vi "Set Protocol Data.vi"(7 "Operation":T1, 8 "error in (no error)":errorcluster, 10 "Protocols.lvlib:Protocol Parent.lvclass":refnum<class "Protocol Parent.lvclass">, 11 "Listener In.lvclass":refnum<class "Listener.lvclass"> caption="Listener") -> (0 "error out":errorcluster, 3 "Listener Out.lvclass":refnum<class "Listener.lvclass">)   [LabVIEW 2019, in "Listener.lvclass"]
uses:
  Listener.lvclass
  Protocol Parent/Protocol Parent.lvclass
  ListenerClassControls/Operation.ctl
  AK TCP/AK TCP.lvclass
  D:/GitRepository/niveristand-instrument-addon-classes/Source/Protocols/TCP/TCP.lvclass
  ListenerClassControls/AK TCP Data Structure.ctl
  ListenerClassControls/Protocol.ctl
  TCP/TCP.lvclass/TCP.ctl
  TCP/TCP.lvclass
  ListenerClassControls/TCP Data Structure.ctl
  UDP/UDP.lvclass
  ListenerClassControls/UDP Data Structure.ctl
  UDP/UDP.lvclass/UDP.ctl
  TCP/Data Access/Read IP Address.vi
  TCP/Data Access/Read Port.vi
  UDP/Data Access/Read Target IP Address.vi
  UDP/Data Access/Read Local Port.vi
  UDP/Data Access/Read Local IP Address.vi
  UDP/Data Access/Read Target Port.vi
  Constants.vi
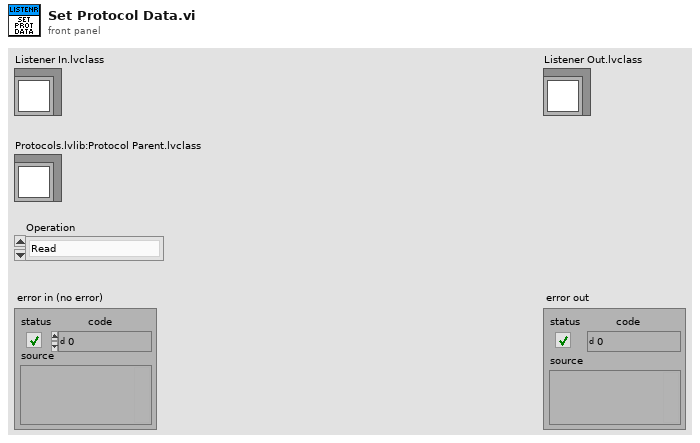
[diagram p1: front panel]
types:
  T1 = typedef "Listener.lvclass/Operation.ctl" = enum16{"Read", "Write"}
  T2 = typedef "Listener.lvclass/Protocol.ctl" = enum16{"RS-XXX", "AK RS-XXX", "VISA", "TCPIP", "AK TCPIP", "UDP", "GPIB ConvBox"}
  T3 = typedef "Listener.lvclass/AK TCP Data Structure.ctl" = cluster{"TCP|IP connection ID":refnum<k5>, "IP Address":string, "Port":u16, "Data":string, "Current Command Code":string}
  T4 = typedef "Listener.lvclass/TCP Data Structure.ctl" = cluster{"TCP|IP connection ID":refnum<k5>, "IP Address":string, "Port":u16, "Data":string}
  T5 = typedef "Listener.lvclass/UDP Data Structure.ctl" = cluster{"UDP connection ID":refnum<k16>, "Local Address":string, "Local Port":u16, "Target IP Address":string, "Target Port":u16, "Data":string}
  T6 = typedef "Protocols.lvlib/Protocol Parent.lvclass/Base Protocol Type.ctl" = enum16{"RS-XXX", "VISA", "TCPIP", "UDP", "GPIB ConvBox"}
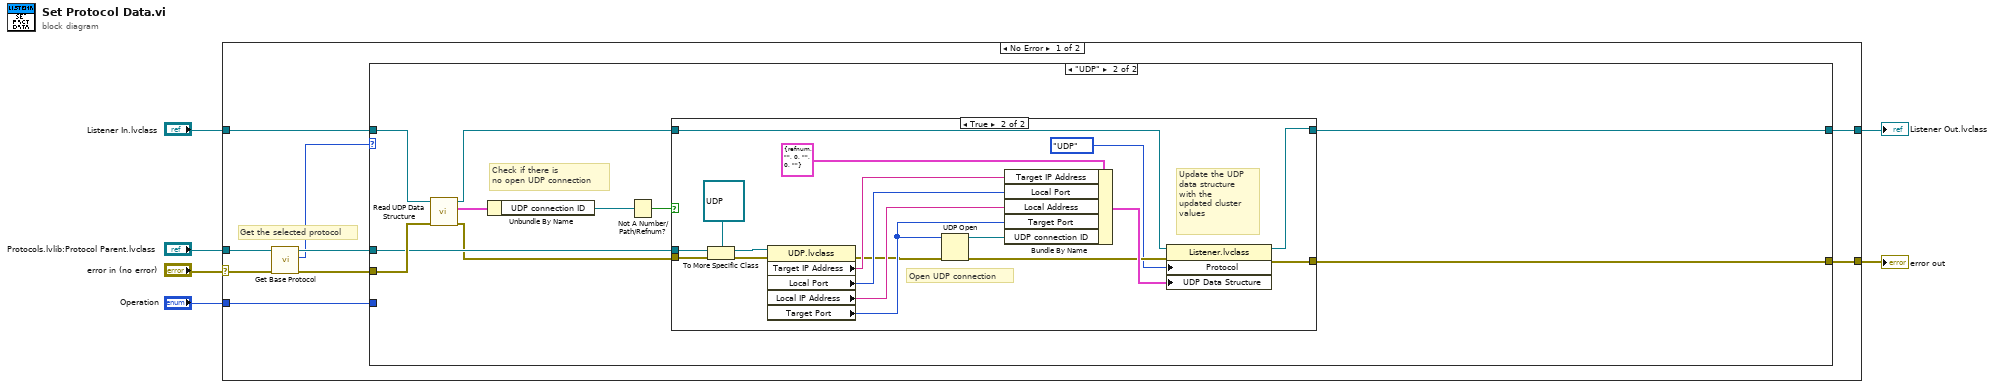
[diagram p0: block diagram]
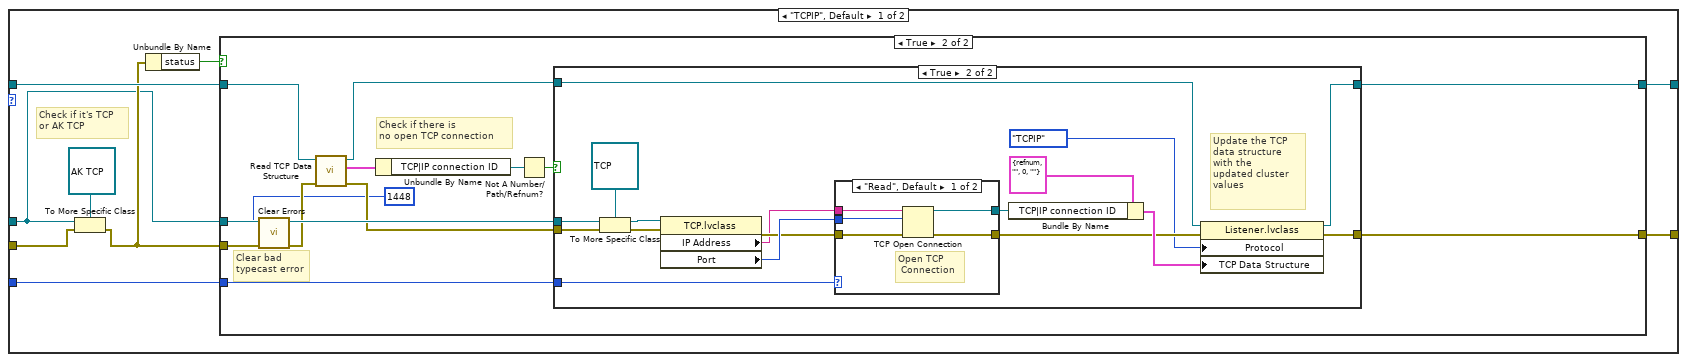
[diagram p2: hidden frame]
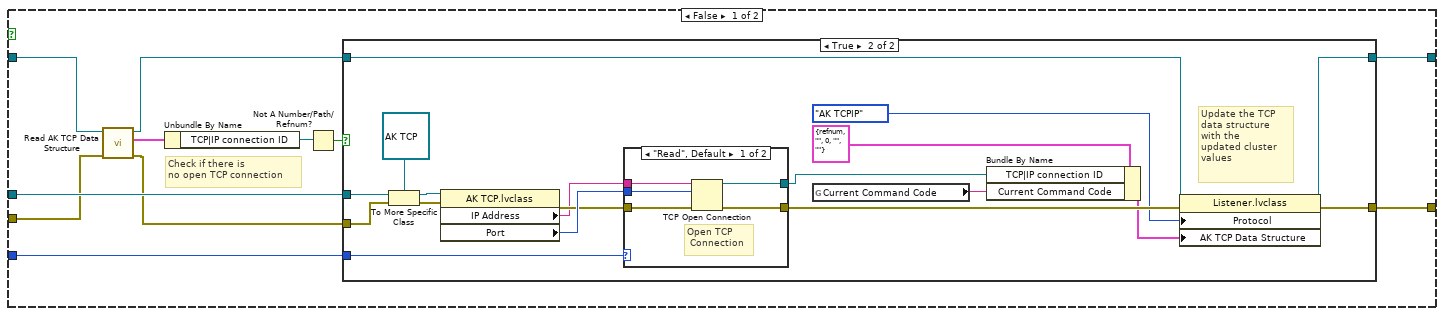
[diagram p3: hidden frame]
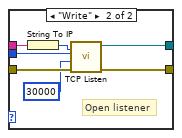
[diagram p5: hidden frame]
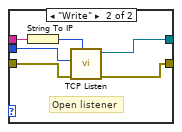
[diagram p7: hidden frame]
diagram:
  n1 = case shown="No Error" "error in (no error)" {
    selector: "error in (no error)" -> [w13 w142]
    tunnel: [w12 w142] -> w5
    tunnel: "Protocols.lvlib:Protocol Parent.lvclass" -> [w14 _]
    tunnel: "Listener In.lvclass" -> [w11 w141]
    tunnel: [w8 w141] -> w2
    tunnel: "Operation" -> [w7 _]
    frame No Error {
      # "Get the selected protocol"
      n2 = call-dynamic "Get Base Protocol.vi"("error in (no error)"=w13, "Protocol Parent in"=w14) -> ("error out"=w10:errorcluster, "Protocol out"=w9:T6, "Protocol Parent out"=w15:refnum<class "Protocol Parent.lvclass">)  [unwired: 7 in]
      n3 = case shown="\"UDP\"" w9 {
        tunnel: w15 -> [w16 w114]
        tunnel: w10 -> [w20 w116]
        tunnel: [w23 w119] -> w12
        tunnel: w11 -> [w22 w115]
        tunnel: [w24 w120] -> w8
        tunnel: w7 -> [w21 _]
        frame "TCPIP", Default {
          # "Check if it's TCP \nor AK TCP"
          n4 = To More Specific Class(target class=refnum<class "AK TCP.lvclass"> refnum ("Protocols.lvlib:AK TCP.lvclass"), reference=w16, error in=w20) -> (error out=w19:errorcluster)  [unwired: 1 out]
          n5 = Unbundle By Name(w19) -> ("status"=w18:bool)
          n6 = case shown="True" w18 {
            tunnel: w16 -> [w35 w80]
            tunnel: [w34 w79] -> w24
            tunnel: [w33 w78] -> w23
            tunnel: w22 -> [w30 w76]
            tunnel: w19 -> [w28 w75]
            tunnel: w21 -> [w31 w70]
            frame False {
              # "Check if there is \nno open TCP connection"
              n7 = call-dynamic "Read AK TCP Data Structure.vi"("error in (no error)"=w28, "Listener in"=w30) -> ("error out"=w27:errorcluster, "TCP|IP Data Structure"=w26:T3, "Listener out"=w29:refnum<class "Listener.lvclass">)  [unwired: 7 in]
              n8 = Unbundle By Name(w26) -> ("TCP|IP connection ID"=w25:refnum<k5>)
              n9 = Not A Number/Path/Refnum?(number/path/refnum=w25) -> (NaN/Path/Refnum?=w32:bool)
              n10 = case shown="True" w32 {
                tunnel: w35 -> [_ w55]
                tunnel: [w37 w52] -> w34
                tunnel: [w36 w51] -> w33
                tunnel: w27 -> [w36 w50]
                tunnel: w29 -> [w37 w49]
                tunnel: w31 -> [_ w48]
                frame False {
                }
                frame True {
                  # "Update the TCP \ndata structure\nwith the\nupdated cluster\nvalues"
                  n11 = To More Specific Class(target class=refnum<class "AK TCP.lvclass"> refnum ("Protocols.lvlib:AK TCP.lvclass"), reference=w55, error in=w50) -> (specific class reference=w54:refnum<class "AK TCP.lvclass">, error out=w53:errorcluster)
                  n12 = property class="AK TCP.lvclass"(reference=w54, error in=w53) -> (error out=w46:errorcluster, "IP Address"=w45:string, "Port"=w47:u16)  [unwired: 1 out]
                  n13 = case shown="\"Read\", Default" w48 {
                    tunnel: w47 -> [w60 w62]
                    tunnel: w46 -> [w59 w67]
                    tunnel: w45 -> [w58 w66]
                    tunnel: [w57 w63] -> w44
                    tunnel: [w56 w64] -> w43
                    frame "Read", Default {
                      # "Open TCP\n Connection"
                      n14 = TCP Open Connection(address=w58, remote port or service name=w60, error in (no error)=w59) -> (connection ID=w56:refnum<k5>, error out=w57:errorcluster)  [unwired: 2 in]
                    }
                    frame "Write" {
                      # "Open listener"
                      n15 = String To IP(1:w66) -> (0:w65:u32)
                      n16 = call <vilib>:"TCP Listen.vi"("net address"=w65, "error in (no error)"=w67, "timeout ms (wait forever: -1)"=30000, "port"=w62) -> ("error out"=w63:errorcluster, "connection ID"=w64:refnum<k5>)  [unwired: 3 in, 3 out]
                    }
                  }
                  n17 = global read "Constants.vi" "Current Command Code"() -> (w38:string)
                  n18 = Bundle By Name(cluster=T3 {"TCP|IP connection ID"=refnum, "IP Address"="", "Port"=0, "Data"="", "Current Command Code"=""} ("TCP|IP Data Structure"), "TCP|IP connection ID"=w43, "Current Command Code"=w38) -> (w40:T3)
                  n19 = property class="Listener.lvclass"(reference=w49, error in=w44, "Protocol"=Protocol."AK TCPIP", "AK TCP Data Structure"=w40) -> (reference out=w52:refnum<class "Listener.lvclass">, error out=w51:errorcluster)
                }
              }
            }
            frame True {
              # "Clear bad \ntypecast error"
              # "Check if there is \nno open TCP connection"
              n20 = call <vilib>:"Clear Errors.vi"("error in (no error)"=w75, "specific error code to clear (0: all)"=1448) -> ("error out"=w69:errorcluster)  [unwired: 4 in, 1 out]
              n21 = call-dynamic "Read TCP Data Structure.vi"("error in (no error)"=w69, "Listener in"=w76) -> ("error out"=w74:errorcluster, "TCP|IP Data Structure"=w73:T4, "Listener out"=w72:refnum<class "Listener.lvclass">)  [unwired: 7 in]
              n22 = Unbundle By Name(w73) -> ("TCP|IP connection ID"=w77:refnum<k5>)
              n23 = Not A Number/Path/Refnum?(number/path/refnum=w77) -> (NaN/Path/Refnum?=w71:bool)
              n24 = case shown="True" w71 {
                tunnel: w80 -> [_ w98]
                tunnel: [w82 w94] -> w79
                tunnel: [w81 w92] -> w78
                tunnel: w74 -> [w81 w91]
                tunnel: w72 -> [w82 w90]
                tunnel: w70 -> [_ w89]
                frame False {
                }
                frame True {
                  # "Update the TCP \ndata structure\nwith the\nupdated cluster\nvalues"
                  n25 = To More Specific Class(target class=refnum<class "TCP.lvclass"> refnum ("Protocols.lvlib:TCP.lvclass"), reference=w98, error in=w91) -> (specific class reference=w97:refnum<class "TCP.lvclass">, error out=w96:errorcluster)
                  n26 = property class="TCP.lvclass"(reference=w97, error in=w96) -> (error out=w87:errorcluster, "IP Address"=w86:string, "Port"=w88:u16)  [unwired: 1 out]
                  n27 = case shown="\"Read\", Default" w89 {
                    tunnel: w88 -> [w104 w109]
                    tunnel: w87 -> [w103 w110]
                    tunnel: w86 -> [w102 w108]
                    tunnel: [w101 w105] -> w85
                    tunnel: [w100 w106] -> w84
                    frame "Read", Default {
                      # "Open TCP\n Connection"
                      n28 = TCP Open Connection(address=w102, remote port or service name=w104, error in (no error)=w103) -> (connection ID=w100:refnum<k5>, error out=w101:errorcluster)  [unwired: 2 in]
                    }
                    frame "Write" {
                      # "Open listener"
                      n29 = String To IP(1:w108) -> (0:w107:u32)
                      n30 = call <vilib>:"TCP Listen.vi"("net address"=w107, "error in (no error)"=w110, "port"=w109) -> ("error out"=w105:errorcluster, "connection ID"=w106:refnum<k5>)  [unwired: 4 in, 3 out]
                    }
                  }
                  n31 = Bundle By Name(cluster=T4 {"TCP|IP connection ID"=refnum, "IP Address"="", "Port"=0, "Data"=""} ("TCP|IP Data Structure"), "TCP|IP connection ID"=w84) -> (w93:T4)
                  n32 = property class="Listener.lvclass"(reference=w90, error in=w85, "Protocol"=Protocol."TCPIP", "TCP Data Structure"=w93) -> (reference out=w94:refnum<class "Listener.lvclass">, error out=w92:errorcluster)
                }
              }
            }
          }
        }
        frame "UDP" {
          # "Check if there is \nno open UDP connection"
          n33 = call-dynamic "Read UDP Data Structure.vi"("error in (no error)"=w116, "Listener in"=w115) -> ("error out"=w112:errorcluster, "UDP Data Structure"=w113:T5, "Listener out"=w111:refnum<class "Listener.lvclass">)  [unwired: 7 in]
          n34 = Unbundle By Name(w113) -> ("UDP connection ID"=w117:refnum<k16>)
          n35 = Not A Number/Path/Refnum?(number/path/refnum=w117) -> (NaN/Path/Refnum?=w118:bool)
          n36 = case shown="True" w118 {
            tunnel: w112 -> [w122 w140]
            tunnel: w114 -> [_ w138]
            tunnel: w111 -> [w121 w132]
            tunnel: [w121 w131] -> w120
            tunnel: [w122 w129] -> w119
            frame False {
            }
            frame True {
              # "Update the UDP \ndata structure\nwith the\nupdated cluster\nvalues"
              # "Open UDP connection"
              n37 = To More Specific Class(target class=refnum<class "UDP.lvclass"> refnum ("Protocols.lvlib:UDP.lvclass"), reference=w138, error in=w140) -> (specific class reference=w128:refnum<class "UDP.lvclass">, error out=w137:errorcluster)
              n38 = property class="UDP.lvclass"(reference=w128, error in=w137) -> (error out=w126:errorcluster, "Target IP Address"=w136:string, "Local Port"=w135:u16, "Local IP Address"=w134:string, "Target Port"=w127:u16)  [unwired: 1 out]
              n39 = UDP Open(8:w126, 11:w127) -> (port=w125:refnum<k16>, 0:w124:errorcluster)  [unwired: 3 in, 1 out]
              n40 = Bundle By Name(cluster=T5 {"UDP connection ID"=refnum, "Local Address"="", "Local Port"=0, "Target IP Address"="", "Target Port"=0, "Data"=""} ("UDP Data Structure"), "Target IP Address"=w136, "Local Port"=w135, "Local Address"=w134, "Target Port"=w127, "UDP connection ID"=w125) -> (w130:T5)
              n41 = property class="Listener.lvclass"(reference=w132, error in=w124, "Protocol"=Protocol."UDP", "UDP Data Structure"=w130) -> (reference out=w131:refnum<class "Listener.lvclass">, error out=w129:errorcluster)
            }
          }
        }
      }
    }
    frame Error {
    }
  }
  "Listener Out.lvclass" <- w2
  "error out" <- w5
